vi "set_x_amplitude.vi"(8 "error in (no error)":errorcluster, 10 "x amplitude":dbl[unit], 11 "TrajectoryTS090820Circular2D in":refnum<class "TrajectoryTS090820Circular2D.lvclass">) -> (0 "error out":errorcluster, 3 "TrajectoryTS090820Circular2D out":refnum<class "TrajectoryTS090820Circular2D.lvclass">)   [LabVIEW 2010, in "TrajectoryTS090820Circular2D.lvclass"]
uses:
  TrajectoryTS090820Circular2D.lvclass
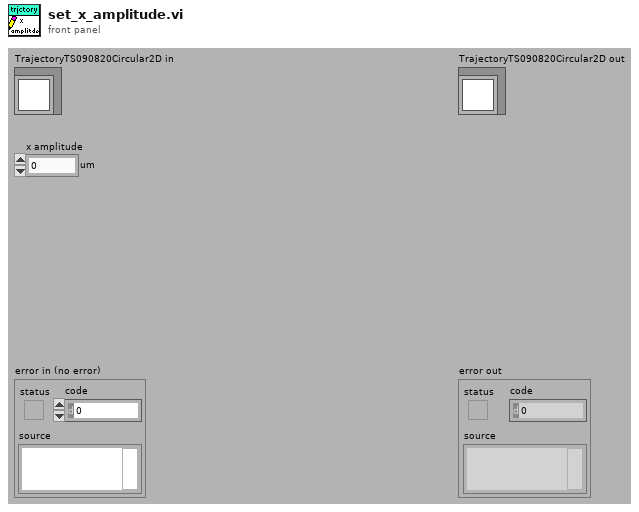
[diagram p1: front panel]
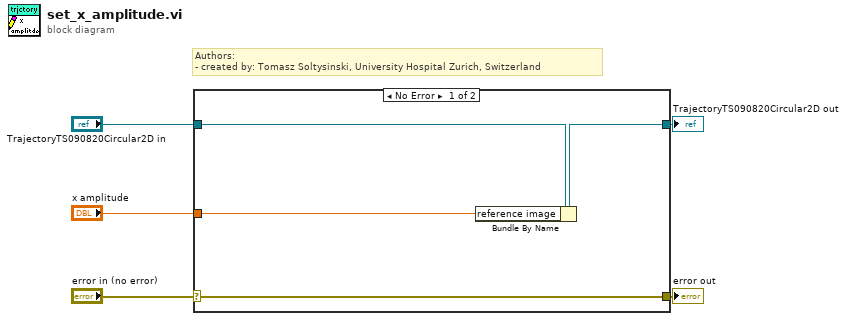
[diagram p0: block diagram]
diagram:
  # "Authors: \n- created by: Tomasz Soltysinski, University Hospital Zurich, Switzerland"
  n1 = case shown="No Error" "error in (no error)" {
    selector: "error in (no error)" -> [w9 w10]
    tunnel: [w9 w10] -> w4
    tunnel: [w7 w11] -> w2
    tunnel: "TrajectoryTS090820Circular2D in" -> [w8 w11]
    tunnel: "x amplitude" -> [w6 _]
    frame No Error {
      n2 = Bundle By Name(cluster=w8, "reference image"=w6) -> (w7:refnum<class "TrajectoryTS090820Circular2D.lvclass">)
    }
    frame Error {
    }
  }
  "error out" <- w4
  "TrajectoryTS090820Circular2D out" <- w2
